vi "Sort Current in Ascending Order.vi"(0 "Current Array in":dbl[](array[numeric])) -> (5 "Sorted?":bool, 6 "Current Array out":dbl[](array[numeric]), 10 "Not ascending/descending order?":bool)   [LabVIEW 2019]
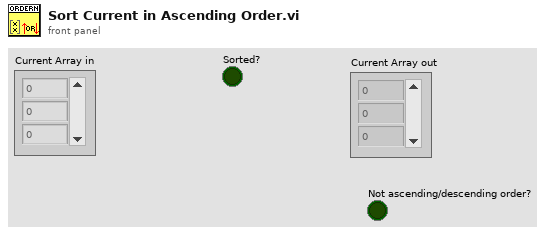
[diagram p1: front panel]
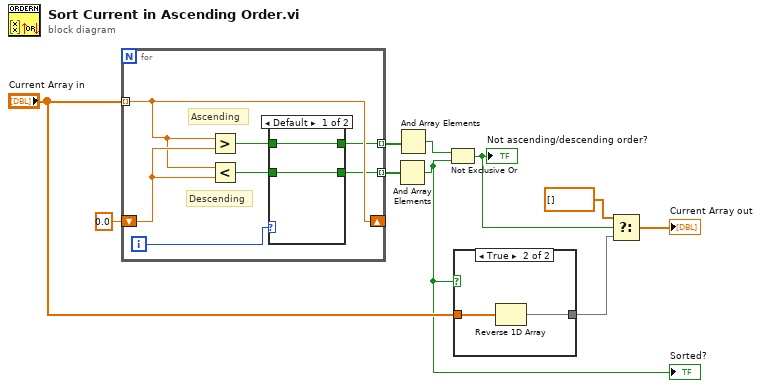
[diagram p0: block diagram]
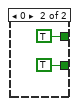
[diagram p3: hidden frame]
diagram:
  n1 = for {
    tunnel: "Current Array in" -> [w16] mode=indexing
    shift-right: [w16] -> _
    shift-left: 0.0 ("Numeric") -> [w17]
    tunnel: [w15] -> w10 mode=indexing
    tunnel: [w13] -> w9 mode=indexing
    i -> [w11]
    # "Descending"
    # "Ascending"
    n2 = Greater?(x=w16, y=w17) -> (0:w14:bool)
    n3 = Less?(x=w16, y=w17) -> (x < y?=w12:bool)
    n4 = case shown="Default" w11 {
      tunnel: [w19 TRUE] -> w15
      tunnel: w14 -> [w19 _]
      tunnel: [w18 TRUE] -> w13
      tunnel: w12 -> [w18 _]
      frame Default {
      }
      frame 0 {
      }
    }
  }
  n5 = And Array Elements(Boolean array=w9) -> (logical AND=w1:bool)
  "Sorted?" <- w1
  n6 = And Array Elements(Boolean array=w10) -> (logical AND=w8:bool)
  n7 = Not Exclusive Or(1:w1, 2:w8) -> (0:w5:bool)
  "Not ascending/descending order?" <- w5
  n8 = case shown="True" w1 {
    tunnel: "Current Array in" -> [w22 w24]
    tunnel: [w22 w23] -> w4
    frame False {
    }
    frame True {
      n9 = Reverse 1D Array(array=w24) -> (reversed array=w23:dbl[])
    }
  }
  n10 = Select(t=dbl[] [], s=w5, f=w4) -> (s? t:f=→"Current Array out":dbl[])
